vi "Main.vi"(11 "Module Admin":refnum<class "Delacor_lib_QMH_Module Admin.lvclass">) -> ()   [LabVIEW 2017, in "SingletonModule.lvlib"]
doc: "This template is based off of the Queued Message Handler design pattern and the Queued Message Handler project template that ships with LabVIEW.\n\nThe main difference is that the queue is private to this module and communication between modules is performed via Broadcast and Request events.\n\nRequest events are wrapped in public API methods and are handled in the Event Handling Loop (EHL) of this VI. Any module can register for Broadcast events sent by this module. The EHL generates messages based on user interface actions.\n\nThe Message Handling Loop (MHL) processes messages generated by the EHL, or by other messages. The messages are string values, so new messages can be added easily to the Message Cases case structure in the MHL. Each message cluster can also provide an optional value for Message Data, which is a variant that can be converted to whatever message-specific data is required.\n_____\nBased on DQMH Project Template 6.1.0.94."
uses:
  SingletonModule.lvlib
  <vilib>/Delacor/Delacor QMH/Libraries/Module Admin_class/Delacor_lib_QMH_Module Admin.lvclass
  Module Data--cluster.ctl
  <vilib>/Delacor/Delacor QMH/Libraries/Message Queue_class/Delacor_lib_QMH_Message Queue.lvclass/Delacor_lib_QMH_Message Queue.ctl
  Stop Argument--cluster.ctl
  <vilib>/Delacor/Delacor QMH/Libraries/Module Admin_class/Delacor_lib_QMH_Module Admin.lvclass/Delacor_lib_QMH_Module Admin.ctl
  Request Method Argument--cluster.ctl
  Request and Wait for Reply Argument--cluster.ctl
  Request and Wait for Reply (Reply Payload)--cluster.ctl
  Round Trip Request Argument--cluster.ctl
  Round Trip Request (Reply Payload)--cluster.ctl
  <vilib>/Utility/miscctls.llb/LVPointTypeDef.ctl
  <vilib>/Delacor/Delacor QMH/Libraries/Message Queue_class/Delacor_lib_QMH_Enqueue Message (Single).vi
  <vilib>/Delacor/Delacor QMH/Libraries/Module Admin_class/Delacor_lib_QMH_Get External Launch.vi
  <vilib>/Utility/error.llb/Error Cluster From Error Code.vi
  <vilib>/ErrorRing/Error Ring.xnode
  <vilib>/Delacor/Delacor QMH/Libraries/Message Queue_class/Delacor_lib_QMH_Message Queue.lvclass
panel:
  out "error out":errorcluster
  out "Status":string
  in  "Simulate MHL Error":bool
  in  "Simulate EHL Error":bool
  # "Other QMH Modules communicate with this Module via its Public API (wrappers for its Request Events).\n\nThis Module communicates with other Modules via its Broadcast Events.\nAny module that wants to get these messages, just registers for this module's Broadcast events."
  # "This template is for the Delacor Modified Queued Message Handler design pattern.\n\nSee the block diagram for more information on how to use this template."
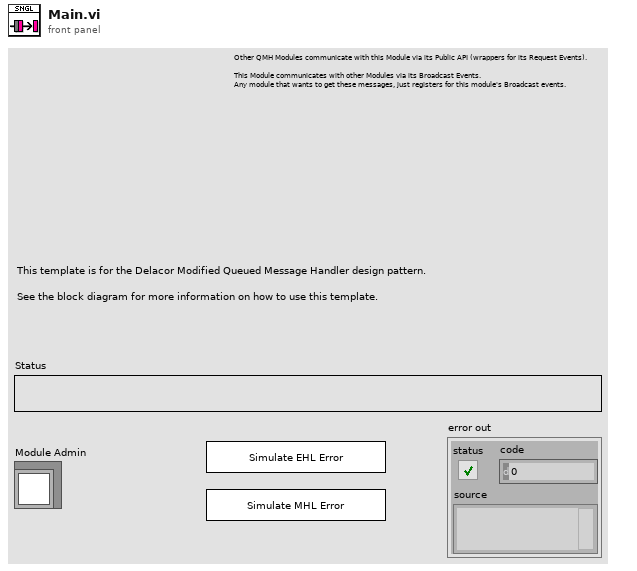
[diagram p1: front panel]
types:
  T1 = typedef "SingletonModule.lvlib/Request Events--cluster.ctl" = cluster{"Stop Module":refnum<user-event>, "Show Panel":refnum<user-event>, "Hide Panel":refnum<user-event>, "Get Module Execution Status":refnum<user-event>, "Show Diagram":refnum<user-event>, "Request Method":refnum<user-event>, "Request and Wait for Reply":refnum<user-event>, "Round Trip Request":refnum<user-event>}
  T2 = typedef "SingletonModule.lvlib/Module Data--cluster.ctl" = cluster{"Status":string, "myData":dbl}
  T3 = enum32{"invalid lock state", "Not Locked", "Locked (No Password)", "Password-protected"}
  T4 = typedef "SingletonModule.lvlib/Stop Argument--cluster.ctl" = cluster{"Origin":string, "Exit via Stop Module Req?":bool, "Wait for Module to stop?":bool}
  T5 = typedef "SingletonModule.lvlib/Request and Wait for Reply Argument--cluster.ctl" = cluster{"Operation":enum16{"Increment", "Decrement"}, "Wait Notifier":refnum<notifier>, "wait for reply":bool}
  T6 = typedef "SingletonModule.lvlib/Round Trip Request Argument--cluster.ctl" = cluster{"Operation":enum16{"Increment", "Decrement"}, "Wait Notifier":refnum<notifier>, "wait for reply":bool}
  T7 = typedef "LVPointTypeDef.ctl" = cluster{"Horizontal":i16, "Vertical":i16}
  T8 = enum32{"Invalid", "Standard", "Closed", "Hidden", "Minimized", "Maximized"}
  T9 = typedef "SingletonModule.lvlib/Request Method Argument--cluster.ctl" = cluster{"myData":dbl}
  T10 = typedef "SingletonModule.lvlib/Request and Wait for Reply (Reply Payload)--cluster.ctl" = cluster{"myData":dbl, "error":errorcluster}
  T11 = typedef "SingletonModule.lvlib/Round Trip Request (Reply Payload)--cluster.ctl" = cluster{"myData":dbl, "error":errorcluster}
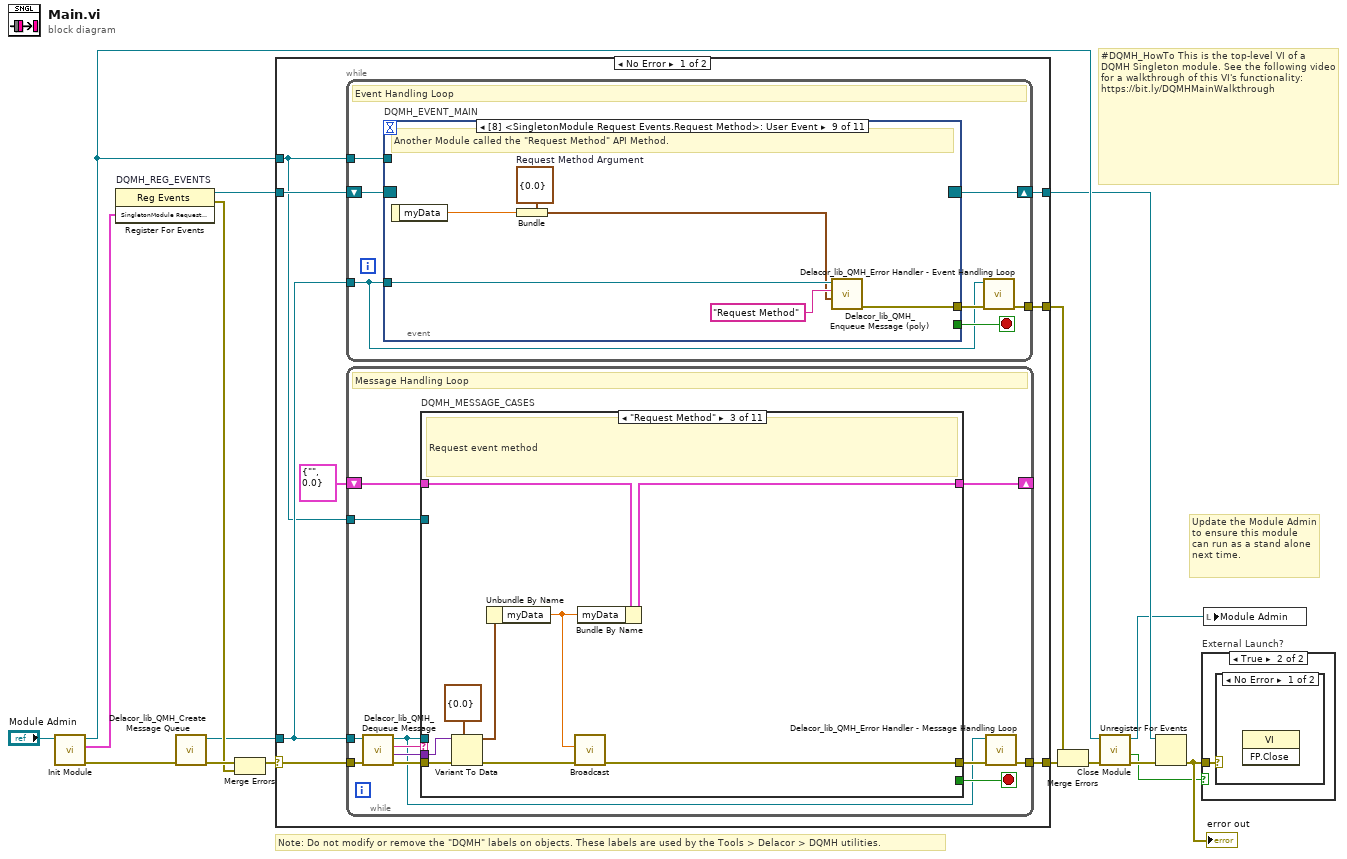
[diagram p0: block diagram]
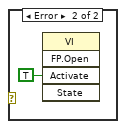
[diagram p3: hidden frame]
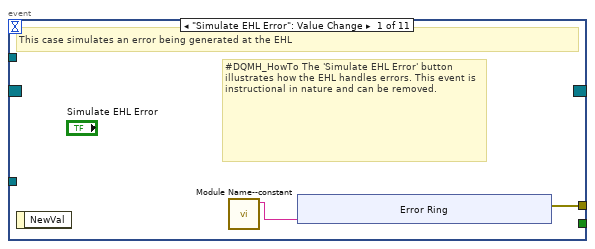
[diagram p4: hidden frame]
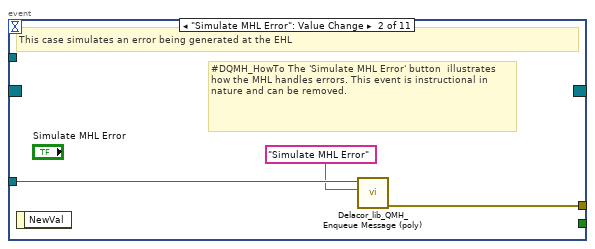
[diagram p5: hidden frame]
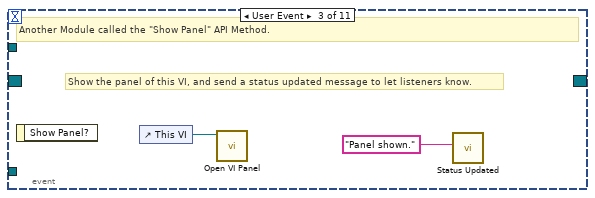
[diagram p6: hidden frame]
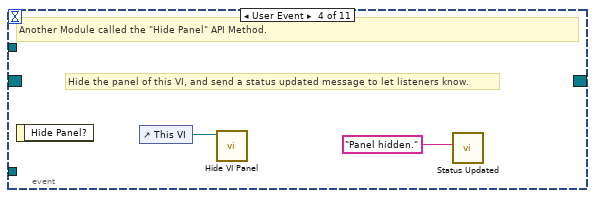
[diagram p7: hidden frame]
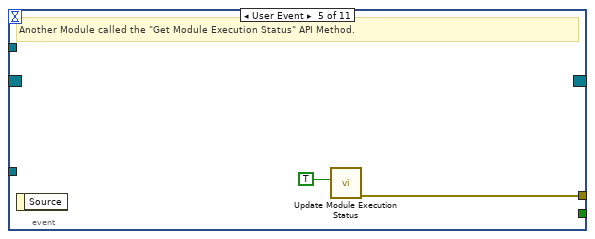
[diagram p8: hidden frame]
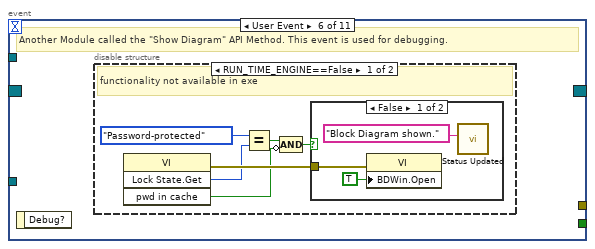
[diagram p9: hidden frame]
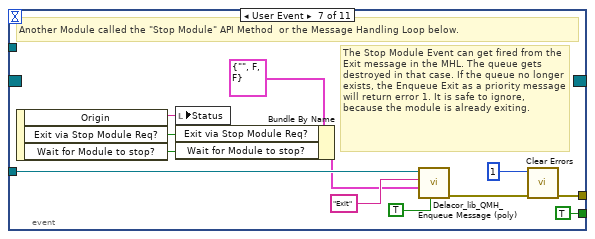
[diagram p12: hidden frame]
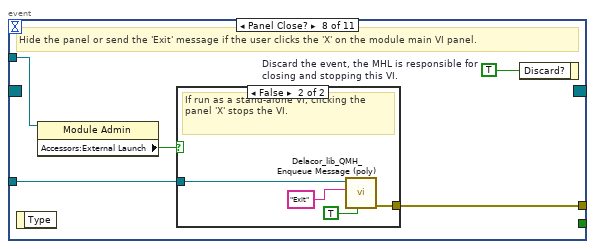
[diagram p13: hidden frame]
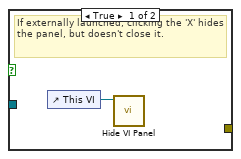
[diagram p14: hidden frame]
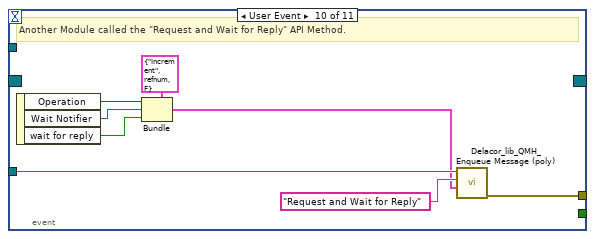
[diagram p15: hidden frame]
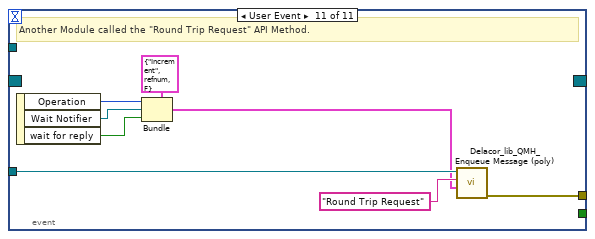
[diagram p16: hidden frame]
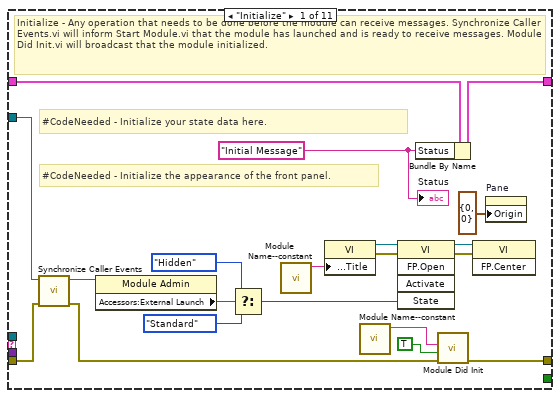
[diagram p17: hidden frame]
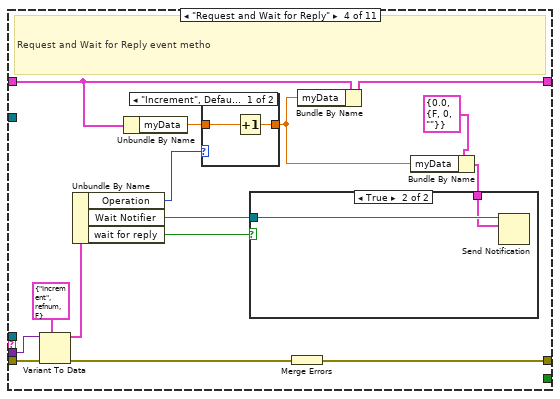
[diagram p19: hidden frame]
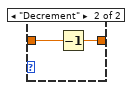
[diagram p20: hidden frame]
diagram:
  # "#DQMH_HowTo This is the top-level VI of a DQMH Singleton module. See the following video for a walkthrough of this VI's functionality: https://bit.ly/DQMHMainWalkthrough"
  # "Note: Do not modify or remove the \"DQMH\" labels on objects. These labels are used by the Tools > Delacor > DQMH utilities."
  # "Update the Module Admin to ensure this module can run as a stand alone next time."
  n1 = call "Init Module.vi"("Singleton Module Admin in"="Module Admin") -> ("error out"=w16:errorcluster, "SingletonModule Request Events"=w5:T1, "Singleton Module Admin out"=w8:refnum<class "Delacor_lib_QMH_Module Admin.lvclass">)  [unwired: 8 in]
  n2 = register-events "DQMH_REG_EVENTS"(w5) -> (reference out=w6:refnum<event-registration>, error out=w9:errorcluster)  [unwired: 2 in]
  n3 = call <vilib>:"Delacor_lib_QMH_Create Message Queue.vi"("error in"=w16) -> ("error out"=w11:errorcluster, "Message Queue"=w4:refnum<class "Delacor_lib_QMH_Message Queue.lvclass">)  [unwired: 9 in]
  n4 = Merge Errors(w11, w9) -> (w10:errorcluster)
  n5 = case shown="No Error" w10 {
    selector: w10 -> [w23 w253]
    tunnel: [w25 w252] -> w17
    tunnel: [w22 w258] -> w7
    tunnel: w6 -> [w20 w258]
    tunnel: w4 -> [w19 w251]
    tunnel: [w24 _] -> w14
    tunnel: w8 -> [w18 w254]
    frame No Error {
      n6 = while {
        tunnel: w19 -> [w26]
        shift-right: [w29] -> w22
        shift-left: w20 -> [w30]
        tunnel: [w31] -> w24
        tunnel: w18 -> [w27]
        stop <- w28 stop-if-true
        # "Event Handling Loop"
        n7 = event "DQMH_EVENT_MAIN" shown="[8] <SingletonModule Request Events.Request Method>: User Event" {
          selector: w30 -> [_ _ _ _ _ _ _ _ _ _ _]
          dyn-events: [_ _ _ _ _ _ _ _ _ _ _] -> w29
          timeout: _ -> [_ _ _ _ _ _ _ _ _ _ _]
          tunnel: [_ _ _ _ _ _ TRUE ("Discard?") _ _ _ _] -> w28
          tunnel: w26 -> [_ w43 _ _ _ _ w67 w74 w87 w95 w103]
          tunnel: [w34 w44 _ _ w50 _ w70 w76 w82 w88 w96] -> w32
          tunnel: w27 -> [_ _ _ _ _ _ _ w73 _ _ _]
          event "Simulate EHL Error": Value Change {
            # "#DQMH_HowTo The 'Simulate EHL Error' button  illustrates how the EHL handles errors. This event is instructional in nature and can be removed."
            # "This case simulates an error being generated at the EHL"
            n8 = event-data() -> ()  [unwired: 1 in, 1 out]
            n9 = call "Module Name--constant.vi"() -> ("Module Name"=w33:string)  [unwired: 11 in]
            n10 = xnode "Error Ring"("parameter 0"=w33) -> ("error out"=w34:errorcluster)
          }
          event "Simulate MHL Error": Value Change {
            # "#DQMH_HowTo The 'Simulate MHL Error' button  illustrates how the MHL handles errors. This event is instructional in nature and can be removed."
            # "This case simulates an error being generated at the EHL"
            n11 = event-data() -> ()  [unwired: 1 in, 1 out]
            n12 = call-poly <vilib>:"Delacor_lib_QMH_Enqueue Message (poly).vi"("Message"="Simulate MHL Error", "Message Queue in"=w43) -> ("error out"=w44:errorcluster)  [unwired: 8 in, 1 out]
          }
          event User Event {
            # "Show the panel of this VI, and send a status updated message to let listeners know."
            # "Another Module called the \"Show Panel\" API Method."
            n13 = event-data() -> ()  [unwired: 1 in, 1 out]
            n14 = control-ref of="This VI"() -> (w46:refnum<vi>)
            n15 = call "Open VI Panel.vi"("VI"=w46) -> ()  [unwired: 10 in, 1 out]
            n16 = call "Status Updated.vi"("Status"="Panel shown." ("format string")) -> ()  [unwired: 10 in, 1 out]
          }
          event User Event {
            # "Hide the panel of this VI, and send a status updated message to let listeners know."
            # "Another Module called the \"Hide Panel\" API Method."
            n17 = event-data() -> ()  [unwired: 1 in, 1 out]
            n18 = control-ref of="This VI"() -> (w48:refnum<vi>)
            n19 = call "Hide VI Panel.vi"("VI"=w48) -> ()  [unwired: 10 in, 1 out]
            n20 = call "Status Updated.vi"("Status"="Panel hidden." ("format string")) -> ()  [unwired: 10 in, 1 out]
          }
          event User Event {
            # "Another Module called the \"Get Module Execution Status\" API Method."
            n21 = event-data() -> ()  [unwired: 1 in, 1 out]
            n22 = call "Update Module Execution Status.vi"("Running?"=TRUE) -> ("error out"=w50:errorcluster)  [unwired: 10 in]
          }
          event User Event {
            # "Another Module called the \"Show Diagram\" API Method. This event is used for debugging."
            n23 = event-data() -> ()  [unwired: 1 in, 1 out]
            n24 = disable-structure shown="RUN_TIME_ENGINE==False" {
              frame condition #0 (active) {
                # "functionality not available in exe"
                n25 = invoke class="VI" method="Lock State.Get"() -> (error out=w56:errorcluster, "Get Lock State"=w55:T3, "pwd in cache"=w52:bool)  [unwired: 4 in, 1 out]
                n26 = Equal?(x=T3."Password-protected", y=w55) -> (x = y?=w53:bool)
                n27 = Compound Arithmetic op=AND(w53, invert w52) -> (w51:bool)
                n28 = case shown="False" w51 {
                  tunnel: w56 -> [w59 _]
                  frame False {
                    n29 = property class="VI"(error in=w59, "BDWin.Open"=TRUE ("Block Diagram Window:Open")) -> ()  [unwired: 1 in, 2 out]
                    n30 = call "Status Updated.vi"("Status"="Block Diagram shown." ("format string")) -> ()  [unwired: 10 in, 1 out]
                  }
                  frame True {
                    # "Password-protected VI, and the password is not in the cache. Do not show the diagram."
                  }
                }
              }
              frame condition #1 {
              }
            }
          }
          event User Event {
            # "The Stop Module Event can get fired from the Exit message in the MHL. The queue gets destroyed in that case. If the queue no longer exists, the Enqueue Exit as a priority message will return error 1. It is safe to ignore, because the module is already exiting."
            # "Another Module called the \"Stop Module\" API Method  or the Message Handling Loop below."
            n31 = event-data() -> ("Origin"=w66:string, "Exit via Stop Module Req?"=w62:bool, "Wait for Module to stop?"=w61:bool)  [unwired: 1 in]
            n32 = local write "Status"(w66) -> ()
            n33 = Bundle By Name(cluster=T4 {"Origin"="", "Exit via Stop Module Req?"=FALSE, "Wait for Module to stop?"=FALSE} ("Stop Argument"), "Exit via Stop Module Req?"=w62, "Wait for Module to stop?"=w61) -> (w60:T4)
            n34 = call-poly <vilib>:"Delacor_lib_QMH_Enqueue Message (poly).vi"("Priority Message? (F)"=TRUE, "Message Data"=w60, "Message"="Exit", "Message Queue in"=w67) -> ("error out"=w71:errorcluster)  [unwired: 6 in, 1 out]
            n35 = call <vilib>:"Clear Errors.vi"("error in (no error)"=w71, "specific error code to clear (0: all)"=1) -> ("error out"=w70:errorcluster)  [unwired: 4 in, 1 out]
          }
          event Panel Close? {
            w75 = TRUE  # Discard the event, the MHL is responsible for closing and stopping this VI.
            # "Hide the panel or send the 'Exit' message if the user clicks the 'X' on the module main VI panel."
            n36 = event-data() -> ()  [unwired: 1 in, 1 out]
            n37 = property class="Module Admin"(reference=w73) -> ("Accessors:External Launch"=w72:bool)  [unwired: 1 in, 2 out]
            n38 = case shown="False" w72 {
              tunnel: w74 -> [_ w80]
              tunnel: [_ w81] -> w76
              frame True {
                # "If externally launched, clicking the 'X' hides the panel, but doesn't close it."
                n39 = control-ref of="This VI"() -> (w77:refnum<vi>)
                n40 = call "Hide VI Panel.vi"("VI"=w77) -> ()  [unwired: 10 in, 1 out]
              }
              frame False {
                # "If run as a stand-alone VI, clicking the panel 'X' stops the VI."
                n41 = call-poly <vilib>:"Delacor_lib_QMH_Enqueue Message (poly).vi"("Priority Message? (F)"=TRUE, "Message"="Exit", "Message Queue in"=w80) -> ("error out"=w81:errorcluster)  [unwired: 7 in, 1 out]
              }
            }
            n42 = event-data("Discard?"=w75) -> ()  [unwired: 1 in, 1 out]
          }
          event User Event {
            w85 = T9 {"myData"=0.0}  # Request Method Argument
            # "Another Module called the \"Request Method\" API Method."
            n43 = event-data() -> ("myData"=w83:dbl)  [unwired: 1 in]
            n44 = Bundle(cluster=w85, "myData"=w83) -> (w84:T9)
            n45 = call-poly <vilib>:"Delacor_lib_QMH_Enqueue Message (poly).vi"("Message Data"=w84, "Message"="Request Method", "Message Queue in"=w87) -> ("error out"=w82:errorcluster)  [unwired: 7 in, 1 out]
          }
          event User Event {
            # "Another Module called the \"Request and Wait for Reply\" API Method."
            n46 = event-data() -> ("Operation"=w91:enum16{"Increment", "Decrement"}, "Wait Notifier"=w90:refnum<notifier>, "wait for reply"=w89:bool)  [unwired: 1 in]
            n47 = Bundle(cluster=T5 {"Operation"=enum."Increment", "Wait Notifier"=refnum, "wait for reply"=FALSE} ("Request and Wait for Reply Argument"), "Operation"=w91, "Wait Notifier"=w90, "wait for reply"=w89) -> (w92:T5)
            n48 = call-poly <vilib>:"Delacor_lib_QMH_Enqueue Message (poly).vi"("Message Data"=w92, "Message"="Request and Wait for Reply", "Message Queue in"=w95) -> ("error out"=w88:errorcluster)  [unwired: 7 in, 1 out]
          }
          event User Event {
            # "Another Module called the \"Round Trip Request\" API Method."
            n49 = event-data() -> ("Operation"=w99:enum16{"Increment", "Decrement"}, "Wait Notifier"=w98:refnum<notifier>, "wait for reply"=w97:bool)  [unwired: 1 in]
            n50 = Bundle(cluster=T6 {"Operation"=enum."Increment", "Wait Notifier"=refnum, "wait for reply"=FALSE} ("Round Trip Request Argument"), "Operation"=w99, "Wait Notifier"=w98, "wait for reply"=w97) -> (w100:T6)
            n51 = call-poly <vilib>:"Delacor_lib_QMH_Enqueue Message (poly).vi"("Message Data"=w100, "Message"="Round Trip Request", "Message Queue in"=w103) -> ("error out"=w96:errorcluster)  [unwired: 7 in, 1 out]
          }
        }
        n52 = call-dynamic "Delacor_lib_QMH_Error Handler - Event Handling Loop.vi"("error in"=w32, "Message Queue in"=w26) -> ("dup error in"=w31:errorcluster)  [unwired: 8 in, 1 out]
      }
      n53 = while {
        tunnel: w19 -> [w106]
        shift-right: [w110] -> _
        shift-left: T2 {"Status"="", "myData"=0.0} ("Data Cluster") -> [w111]
        tunnel: w23 -> [w114]
        tunnel: [w112] -> w25
        tunnel: w18 -> [w104]
        stop <- w109 stop-if-true
        # "Message Handling Loop"
        n54 = call-dynamic "Delacor_lib_QMH_Dequeue Message.vi"("error in"=w114, "Message Queue in"=w106) -> ("error out"=w113:errorcluster, "Message Data"=w107:variant, "Message"=w108:string, "Message Queue out"=w105:refnum<class "Delacor_lib_QMH_Message Queue.lvclass">)  [unwired: 6 in]
        n55 = case "DQMH_MESSAGE_CASES" shown="\"Request Method\"" w108 {
          selector: w108 -> [_ _ _ _ _ _ _ _ _ _ w238]
          tunnel: w105 -> [_ _ _ _ _ _ _ _ w208 w230 _]
          tunnel: w113 -> [w133 w137 w146 w161 w182 w191 w193 w198 w215 w236 w240]
          tunnel: [w131 w137 w138 w152 w173 w190 w193 w197 w211 w233 w241] -> w115
          tunnel: w111 -> [w122 w136 w142 w151 w172 w189 w192 w195 w210 w229 w239]
          tunnel: [w121 w136 w141 w148 w169 w189 w192 w195 w210 w229 w239] -> w110
          tunnel: [_ _ _ _ _ _ _ _ _ w228 _] -> w109
          tunnel: w107 -> [_ _ w145 w159 w180 _ _ _ w209 w227 _]
          tunnel: w104 -> [w123 _ _ _ _ _ _ _ w207 w222 _]
          frame "Initialize" {
            w117 = "Initial Message" ("Initial Message")
            # "#CodeNeeded - Initialize the appearance of the front panel."
            # "#CodeNeeded - Initialize your state data here."
            # "Initialize - Any operation that needs to be done before the module can receive messages. Synchronize Caller Events.vi will inform Start Module.vi that the module has launched and is ready to receive messages. Module Did Init.vi will broadcast that the module initialized."
            n56 = call "Synchronize Caller Events.vi"("error in (no error)"=w133, "Singleton Module Admin in"=w123) -> ("error out"=w132:errorcluster, "Singleton Module Admin out"=w118:refnum<class "Delacor_lib_QMH_Module Admin.lvclass">)  [unwired: 8 in]
            n57 = property class="Module Admin"(reference=w118) -> ("Accessors:External Launch"=w127:bool)  [unwired: 1 in, 2 out]
            n58 = Select(t=T8."Hidden" ("State"), s=w127, f=T8."Standard" ("State")) -> (s? t:f=w124:T8)
            n59 = call "Module Name--constant.vi"() -> ("Module Name"=w130:string)  [unwired: 11 in]
            n60 = property class="VI"("Front Panel.Title"=w130) -> (reference out=w129:refnum<vi>, error out=w135:errorcluster)  [unwired: 2 in]
            n61 = call "Module Name--constant.vi"() -> ("Module Name"=w119:string)  [unwired: 11 in]
            n62 = invoke class="VI" method="FP.Open"(reference=w129, error in=w135, "State"=w124) -> (reference out=w128:refnum<vi>, error out=w134:errorcluster)  [unwired: 2 in, 3 out]
            n63 = Bundle By Name(cluster=w122, "Status"=w117) -> (w121:T2)
            n64 = call "Module Did Init.vi"("error in (no error)"=w132, "Initialized?"=TRUE, "Origin"=w119) -> ("error out"=w131:errorcluster)  [unwired: 8 in]
            n65 = invoke class="VI" method="FP.Center"(reference=w128, error in=w134) -> ()  [unwired: 1 in, 3 out]
            n66 = property on="Pane" class="Pane"("Origin"=T7 {"Horizontal"=0, "Vertical"=0}) -> ()  [unwired: 2 in, 2 out]
            "Status" <- w117
          }
          frame "---Module Specific---" {
            # "Separator -- The following cases handle messages specific to this Module."
          }
          frame "Request Method" {
            # "Request event method"
            n67 = Variant To Data(error in=w146, type=T9 {"myData"=0.0} ("Request Method Argument"), Variant=w145) -> (data=w143:T9, error out=w139:errorcluster)
            n68 = Unbundle By Name(w143) -> ("myData"=w140:dbl)
            n69 = call "Broadcast.vi"("error in"=w139, "myData"=w140) -> ("error out"=w138:errorcluster)  [unwired: 9 in]
            n70 = Bundle By Name(cluster=w142, "myData"=w140) -> (w141:T2)
          }
          frame "Request and Wait for Reply" {
            # "Request and Wait for Reply event metho"
            n71 = Variant To Data(error in=w161, type=T5 {"Operation"=enum."Increment", "Wait Notifier"=refnum, "wait for reply"=FALSE} ("Request and Wait for Reply Argument"), Variant=w159) -> (data=w157:T5, error out=w160:errorcluster)
            n72 = Unbundle By Name(w157) -> ("Operation"=w150:enum16{"Increment", "Decrement"}, "Wait Notifier"=w156:refnum<notifier>, "wait for reply"=w155:bool)
            n73 = Unbundle By Name(w151) -> ("myData"=w149:dbl)
            n74 = case shown="\"Increment\", Default" w150 {
              tunnel: w149 -> [w163 w165]
              tunnel: [w162 w164] -> w147
              frame "Increment", Default {
                n75 = Increment(x=w163) -> (x+1=w162:dbl)
              }
              frame "Decrement" {
                n76 = Decrement(x=w165) -> (x-1=w164:dbl)
              }
            }
            n77 = Merge Errors(w160) -> (w152:errorcluster)
            n78 = Bundle By Name(cluster=w151, "myData"=w147) -> (w148:T2)
            n79 = Bundle By Name(cluster=T10 {"myData"=0.0, "error"={"status"=FALSE, "code"=0, "source"=""}} ("Request and Wait for Reply (Reply Payload)"), "myData"=w147) -> (w154:T10)
            n80 = case shown="True" w155 {
              tunnel: w156 -> [_ w167]
              tunnel: w154 -> [_ w166]
              frame False {
              }
              frame True {
                n81 = Send Notification(notification=w166, notifier=w167) -> ()  [unwired: 1 in, 2 out]
              }
            }
          }
          frame "Round Trip Request" {
            # "Round Trip event method"
            n82 = Variant To Data(error in=w182, type=T6 {"Operation"=enum."Increment", "Wait Notifier"=refnum, "wait for reply"=FALSE} ("Round Trip Request Argument"), Variant=w180) -> (data=w178:T6, error out=w181:errorcluster)
            n83 = Unbundle By Name(w178) -> ("Operation"=w171:enum16{"Increment", "Decrement"}, "Wait Notifier"=w177:refnum<notifier>, "wait for reply"=w176:bool)
            n84 = Unbundle By Name(w172) -> ("myData"=w170:dbl)
            n85 = case shown="\"Increment\", Default" w171 {
              tunnel: w170 -> [w184 w186]
              tunnel: [w183 w185] -> w168
              frame "Increment", Default {
                n86 = Increment(x=w184) -> (x+1=w183:dbl)
              }
              frame "Decrement" {
                n87 = Decrement(x=w186) -> (x-1=w185:dbl)
              }
            }
            n88 = Merge Errors(w181) -> (w173:errorcluster)
            n89 = Bundle By Name(cluster=w172, "myData"=w168) -> (w169:T2)
            n90 = Bundle By Name(cluster=T11 {"myData"=0.0, "error"={"status"=FALSE, "code"=0, "source"=""}} ("Round Trip Request (Reply Payload)"), "myData"=w168) -> (w175:T11)
            n91 = case shown="True" w176 {
              tunnel: w177 -> [_ w188]
              tunnel: w175 -> [_ w187]
              frame False {
              }
              frame True {
                n92 = Send Notification(notification=w187, notifier=w188) -> ()  [unwired: 1 in, 2 out]
              }
            }
            n93 = call "Round Trip Broadcast.vi"("Reply Payload"=w175) -> ()  [unwired: 10 in, 1 out]
          }
          frame "---Copy This Frame---" {
            # "Duplicate this frame when creating new messages.  Change this comment in the duplicated frame to describe this message."
            n94 = Merge Errors(w191) -> (w190:errorcluster)
          }
          frame "---Exit and Error Handling---" {
            # "Separator - The following cases handle errors and exit messages."
          }
          frame "Simulate MHL Error" {
            # "#DQMH_HowTo The 'Simulate MHL Error' button  illustrates how the MHL handles errors. This event is instructional in nature and can be removed."
            # "Simulate an error occurring at the MHL"
            n95 = call "Module Name--constant.vi"() -> ("Module Name"=w194:string)  [unwired: 11 in]
            n96 = xnode "Error Ring"("parameter 0"=w194) -> ("error out"=w196:errorcluster)
            n97 = Merge Errors(w198, w196) -> (w197:errorcluster)
          }
          frame "Error" {
            # "#CodeRecommended - If you ever change the name of this \"Error\" message, you'll need to update the name in the Check Loop Error.vi as well."
            # "#CodeRecommended - If the module is running in standalone mode (External Launch = FALSE), this code will pop up an error dialog and call the 'Exit' message if an error occurs. Add more fine-grained error handling here."
            # "Error - Check the error message data and respond accordingly. This message is sent by the \"Error Handler\" VIs at the end of each loop in this application."
            n98 = property class="Module Admin"(reference=w207) -> ("Accessors:External Launch"=w206:bool)  [unwired: 1 in, 2 out]
            n99 = Variant To Data(error in=w215, type=errorcluster {"status"=FALSE, "code"=0, "source"=""} ("error constant"), Variant=w209) -> (data=w216:errorcluster, error out=w213:errorcluster)
            n100 = call "Error Reported.vi"("Error"=w216) -> ()  [unwired: 10 in, 1 out]
            n101 = case shown="False" w206 {
              tunnel: [w221 _] -> w212
              tunnel: w208 -> [w219 _]
              tunnel: w216 -> [w220 _]
              frame False {
                # "If the module is running standalone, then pop up an error dialog and call the \"Exit\" message."
                n102 = call <vilib>:"Simple Error Handler.vi"("error in (no error)"=w220) -> ()  [unwired: 4 in, 5 out]
                n103 = call-poly <vilib>:"Delacor_lib_QMH_Enqueue Message (poly).vi"("Priority Message? (F)"=TRUE, "Message"="Exit", "Message Queue in"=w219) -> ("error out"=w221:errorcluster)  [unwired: 7 in, 1 out]
              }
              frame True {
                # "If the module was launched externally, calling the Error Reported broadcast VI is the only action performed by the \"Error\" message. The module's caller can then process the error appropriately."
              }
            }
            n104 = Merge Errors(w213, w212) -> (w211:errorcluster)
            n105 = local write "error out"(w211) -> ()
          }
          frame "Exit" {
            w226 = 91  # 91: not all Exit messages will have an argument
            w228 = TRUE  # Stop the VI
            # "Release the message queue reference"
            # "#CodeNeeded - Add any required cleanup code here"
            # "Exit - Exit the application."
            n106 = Variant To Data(error in=w236, type=T4 {"Origin"="", "Exit via Stop Module Req?"=FALSE, "Wait for Module to stop?"=FALSE} ("Stop Argument"), Variant=w227) -> (data=w224:T4, error out=w232:errorcluster)
            n107 = call <vilib>:"Clear Errors.vi"("error in (no error)"=w232, "specific error code to clear (0: all)"=w226) -> ("error out"=w235:errorcluster)  [unwired: 4 in, 1 out]
            n108 = control-ref of="This VI"() -> (w223:refnum<vi>)
            n109 = call-dynamic "Delacor_lib_QMH_Release Message Queue.vi"("error in"=w235, "Message Queue"=w230) -> ("error out"=w234:errorcluster)  [unwired: 9 in]
            n110 = call "Handle Exit.vi"("Stop Argument"=w224, "Admin in"=w222, "VI reference"=w223) -> ("error out"=w231:errorcluster)  [unwired: 7 in, 1 out]
            n111 = Merge Errors(w234, w231) -> (w233:errorcluster)
          }
          frame Default {
            # "'Default' case only runs if there is a message that isn't defined in any of the other cases.  Output a programming error."
            n112 = call "Module Name--constant.vi"() -> ("Module Name"=w237:string)  [unwired: 11 in]
            n113 = xnode "Error Ring"("parameter 0"=w238, "parameter 1"=w237) -> ("error out"=w242:errorcluster)
            n114 = Merge Errors(w240, w242) -> (w241:errorcluster)
          }
        }
        n115 = call-dynamic "Delacor_lib_QMH_Error Handler - Message Handling Loop.vi"("error in"=w115, "Message Queue in"=w105) -> ("dup error in"=w112:errorcluster)  [unwired: 8 in, 1 out]
      }
    }
    frame Error {
      # "Synchronize Caller Events.vi will inform Start Module.vi that the module has launched and will let the code calling Start Module.vi register for broadcasts and would permit the caller receive the broadcast that an error occurred at launch time."
      n116 = call-dynamic "Delacor_lib_QMH_Release Message Queue.vi"("error in"=w253, "Message Queue"=w251) -> ("error out"=w252:errorcluster)  [unwired: 9 in]
      n117 = call "Synchronize Caller Events.vi"("Singleton Module Admin in"=w254) -> ("error out"=w259:errorcluster)  [unwired: 9 in, 1 out]
      n118 = call "Module Name--constant.vi"() -> ("Module Name"=w257:string)  [unwired: 11 in]
      n119 = Format Into String(format string="An error occurred during initialization. %s is no longer running.", w257) -> (resulting string=w255:string)  [unwired: 2 in, 1 out]
      n120 = Merge Errors(w252, w259) -> (w260:errorcluster)
      n121 = call "Error Reported.vi"("Additional Information"=w255, "Error"=w260) -> ()  [unwired: 9 in, 1 out]
    }
  }
  n122 = Merge Errors(w14, w17) -> (w13:errorcluster)
  n123 = call "Close Module.vi"("error in (no error)"=w13, "Module Admin in"=w8) -> ("error out"=w15:errorcluster, "External Launch"=w1:bool, "Module Admin out"=w2:refnum<class "Delacor_lib_QMH_Module Admin.lvclass">)  [unwired: 7 in]
  n124 = Unregister For Events(event registration refnum=w7, error in=w15) -> (error out=w12:errorcluster)
  "error out" <- w12
  n125 = case "External Launch?" shown="True" w1 {
    tunnel: w12 -> [_ w261]
    frame False {
    }
    frame True {
      n126 = case shown="No Error" w261 {
        frame No Error {
          n127 = invoke class="VI" method="FP.Close"() -> ()  [unwired: 3 in, 3 out]
        }
        frame Error {
          n128 = invoke class="VI" method="FP.Open"("Activate"=TRUE ("Activate?")) -> ()  [unwired: 4 in, 5 out]
        }
      }
    }
  }
  n129 = local write "Module Admin"(w2) -> ()
